vi "TelemetryLogger.vi"(6 "Time Stamp":timestamp, 9 "Error In":errorcluster, 10 "Data":variant, 11 "Sensor:Reading":string) -> (1 "Error Out":errorcluster)   [LabVIEW 2017]
uses:
  Type Defs/telemetryReading.ctl
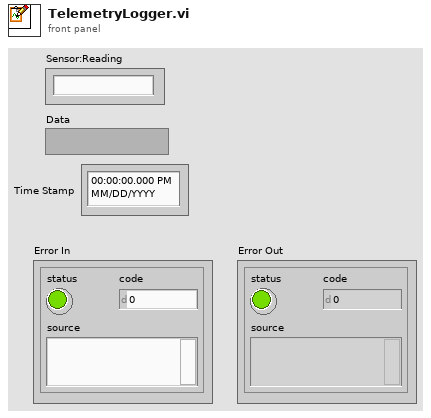
[diagram p1: front panel]
types:
  T1 = typedef "telemetryReading.ctl" = cluster{"Sensor:Reading":string, "Data":variant, "Time Stamp":timestamp}
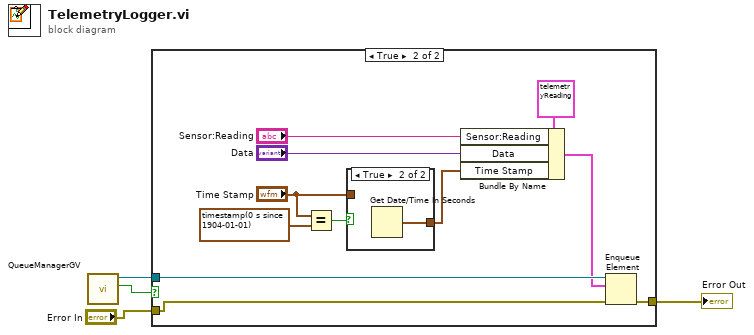
[diagram p0: block diagram]
diagram:
  n1 = call "QueueManagerGV.vi"() -> ("Logging"=w3:bool, "Queue"=w4:refnum<queue>)  [unwired: 10 in]
  n2 = case shown="True" w3 {
    tunnel: w4 -> [_ w9]
    tunnel: "Error In" -> [w5 w7]
    tunnel: [w5 w6] -> w1
    frame False {
    }
    frame True {
      n3 = Equal?(x="Time Stamp", y=timestamp(0 s since 1904-01-01) ("Time Stamp")) -> (x = y?=w13:bool)
      n4 = case shown="True" w13 {
        tunnel: [w17 w18] -> w11
        tunnel: "Time Stamp" -> [w17 _]
        frame False {
        }
        frame True {
          n5 = Get Date/Time In Seconds() -> (seconds since 1Jan1904=w18:timestamp)
        }
      }
      n6 = Bundle By Name(cluster=T1 {"Sensor:Reading"="", "Data"=variant, "Time Stamp"=timestamp(3584563538.456057 s since 1904-01-01)} ("Telemetry Reading"), "Sensor:Reading"="Sensor:Reading", "Data"="Data", "Time Stamp"=w11) -> (w8:T1)
      n7 = Enqueue Element(queue=w9, element=w8, error in (no error)=w7) -> (error out=w6:errorcluster)  [unwired: 1 in, 2 out]
    }
  }
  "Error Out" <- w1
